vi "Calculate I2C.vi"(8 "error in (no error)":errorcluster, 11 "Simulation in":refnum<class "Simulation.lvclass">) -> (0 "error out":errorcluster, 3 "Simulation out":refnum<class "Simulation.lvclass">)   [LabVIEW 2020, in "I2C Storage.lvlib" / "Simulation.lvclass"]
uses:
  Simulation.lvclass
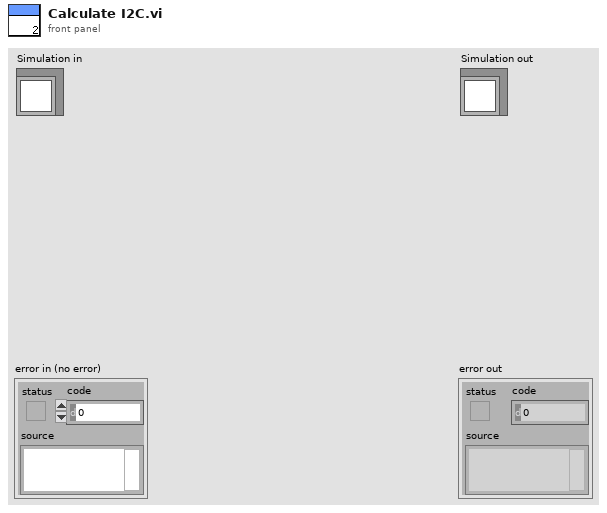
[diagram p1: front panel]
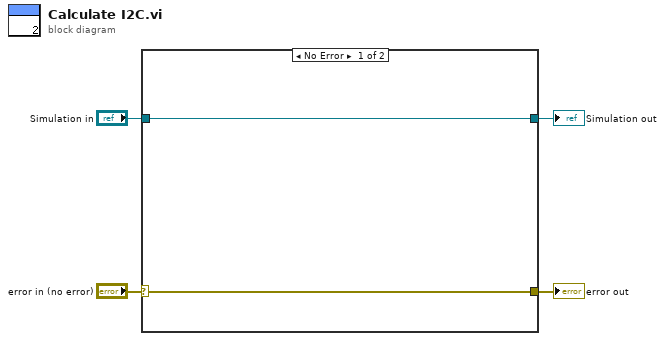
[diagram p0: block diagram]
diagram:
  n1 = case shown="No Error" "error in (no error)" {
    selector: "error in (no error)" -> [w5 w8]
    tunnel: [w6 w7] -> w3
    tunnel: "Simulation in" -> [w6 w7]
    tunnel: [w5 w8] -> w1
    frame No Error {
    }
    frame Error {
      # "Error Found."
    }
  }
  "error out" <- w1
  "Simulation out" <- w3
